vi "time-and-forfunctions.vi"() -> ()   [LabVIEW 2015]
uses:
  <vilib>/Utility/miscctls.llb/LVDateTimeRec.ctl
panel:
  out "date/time string":string
  out "Array":dbl[](array[numeric])
  in  "Tab Control":enum32{"Num to Date Stamp", "Page 2"}(tab)
  in  "number":dbl
  out "time stamp":timestamp
  out "time string":string
  out "date string":string
  out "date time rec":T1
  in  "stop":bool
  out "current time":timestamp
  out "Time Stamp":timestamp=timestamp(3646962314 s since 1904-01-01)
  in  "Ring":u16(ring) items=["Ver hora actual"=0, "Desglosar hora actual"=4, "Third"=42]
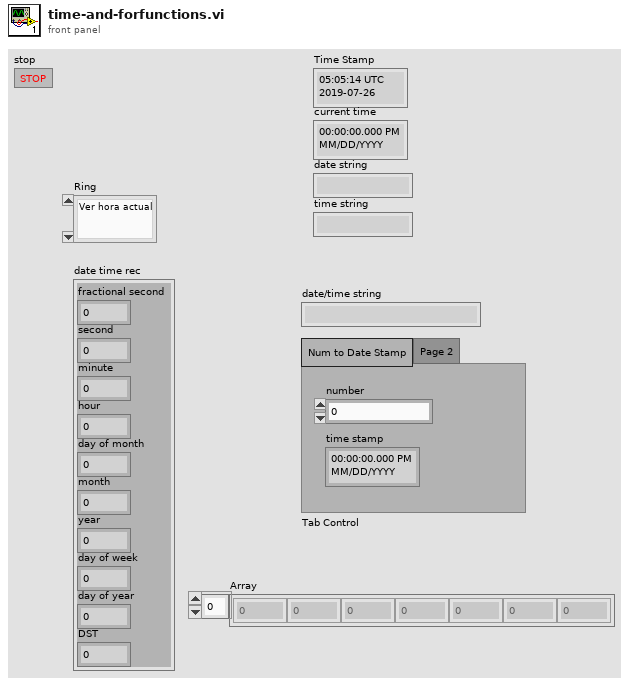
[diagram p1: front panel]
types:
  T1 = typedef "LVDateTimeRec.ctl" = cluster{"fractional second":dbl, "second":i32, "minute":i32, "hour":i32, "day of month":i32, "month":i32, "year":i32, "day of week":i32, "day of year":i32, "DST":i32}
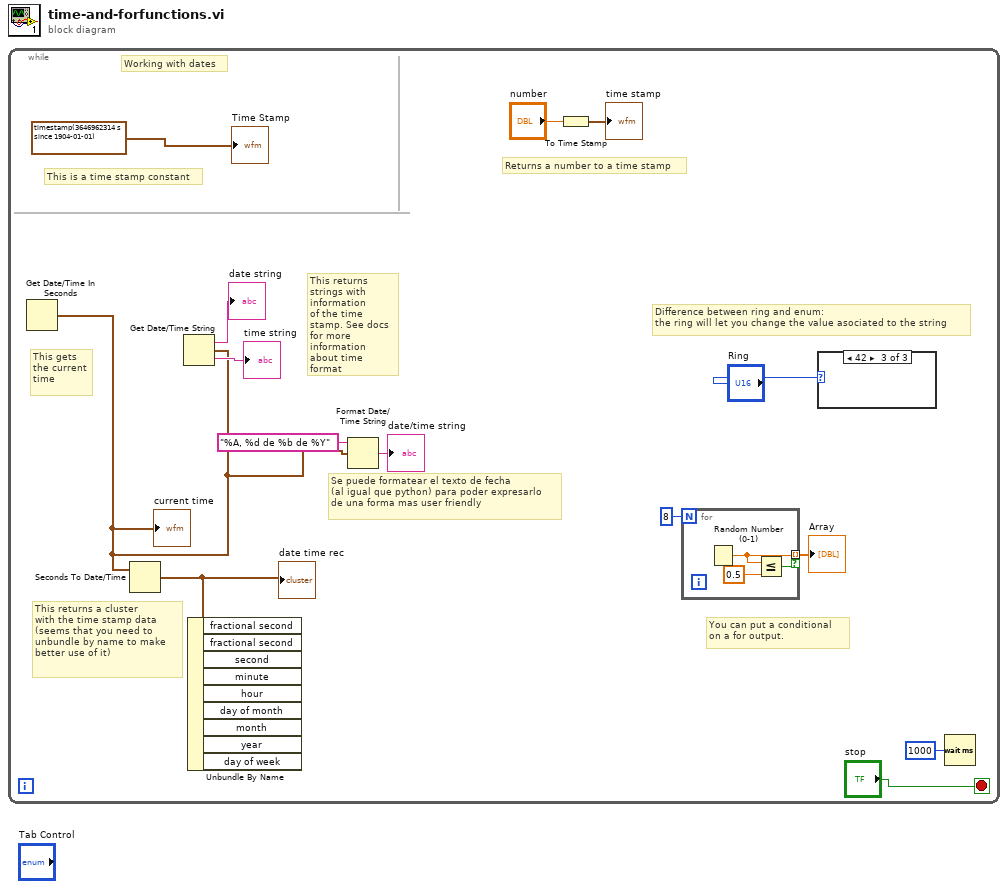
[diagram p0: block diagram]
diagram:
  n1 = while {
    stop <- "stop" stop-if-true
    # "Se puede formatear el texto de fecha\n(al igual que python) para poder expresarlo \nde una forma mas user friendly"
    # "You can put a conditional \non a for output."
    # "Returns a number to a time stamp"
    # "This returns strings with information \nof the time stamp. See docs for more information\nabout time format"
    # "This is a time stamp constant"
    # "This returns a cluster\nwith the time stamp data\n(seems that you need to\nunbundle by name to make\nbetter use of it)"
    # "This gets\nthe current\ntime"
    # "Working with dates"
    # "Difference between ring and enum:\nthe ring will let you change the value asociated to the string"
    n2 = Get Date/Time In Seconds() -> (seconds since 1Jan1904=w3:timestamp)
    "current time" <- w3
    n3 = Seconds To Date/Time(time stamp (now)=w3) -> (date time rec=w10:T1)  [unwired: 1 in]
    "date time rec" <- w10
    n4 = Get Date/Time String(seconds (now)=w3) -> (date string=→"date string":string, time string=→"time string":string)  [unwired: 2 in]
    n5 = Unbundle By Name(w10) -> ()  [unwired: 9 out]
    n6 = Format Date/Time String(time format string (%c)="%A, %d de %b de %Y", seconds (now)=w3) -> (date/time string=→"date/time string":string)  [unwired: 1 in]
    n7 = To Time Stamp(1:"number") -> (0:→"time stamp":timestamp)
    n8 = for {
      N: 8 -> [_]
      tunnel: [w16] -> w4 mode=indexing if=w17
      n9 = Random Number (0-1)() -> (number: 0 to 1=w16:dbl)
      n10 = Less Or Equal?(x=w16, y=0.5) -> (x <= y?=w17:bool)
    }
    "Array" <- w4
    n11 = case shown="42" "Ring" {
      frame 0, Default {
      }
      frame 4 {
      }
      frame 42 {
      }
    }
    n12 = Wait (ms)(milliseconds to wait=u32 1000) -> ()  [unwired: 1 out]
    "Time Stamp" <- timestamp(3646962314 s since 1904-01-01)
  }
